vi "Thread.Get Runnable.vi"(11 "Thread in":refnum<class "Thread.lvclass">) -> (2 "Runnable":refnum<class "Runnable.lvclass">, 3 "Thread out":refnum<class "Thread.lvclass">)   [LabVIEW 2016, in "Thread.lvclass"]
uses:
  Thread.lvclass
  Runnable.lvclass
  Thread.lvclass/Thread.ctl
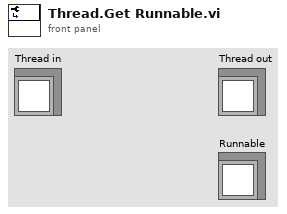
[diagram p1: front panel]
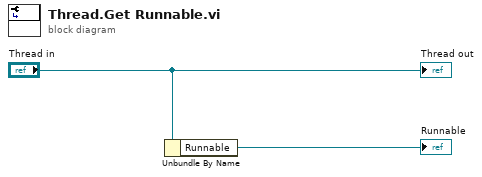
[diagram p0: block diagram]
diagram:
  n1 = Unbundle By Name("Thread in") -> ("Runnable"=→"Runnable":refnum<class "Runnable.lvclass">)
  "Thread out" <- "Thread in"
